vi "导出参数设置3.0.vi"(10 "输入":T1, 11 "路径":path) -> ()   [LabVIEW 2016]
uses:
  <vilib>/Utility/config.llb/Write Key (String).vi
  <vilib>/Utility/config.llb/Write Key (Double).vi
  <vilib>/Utility/config.llb/NI_LVConfig.lvlib
panel:
  in  "ESC":bool
  in  "OK":bool
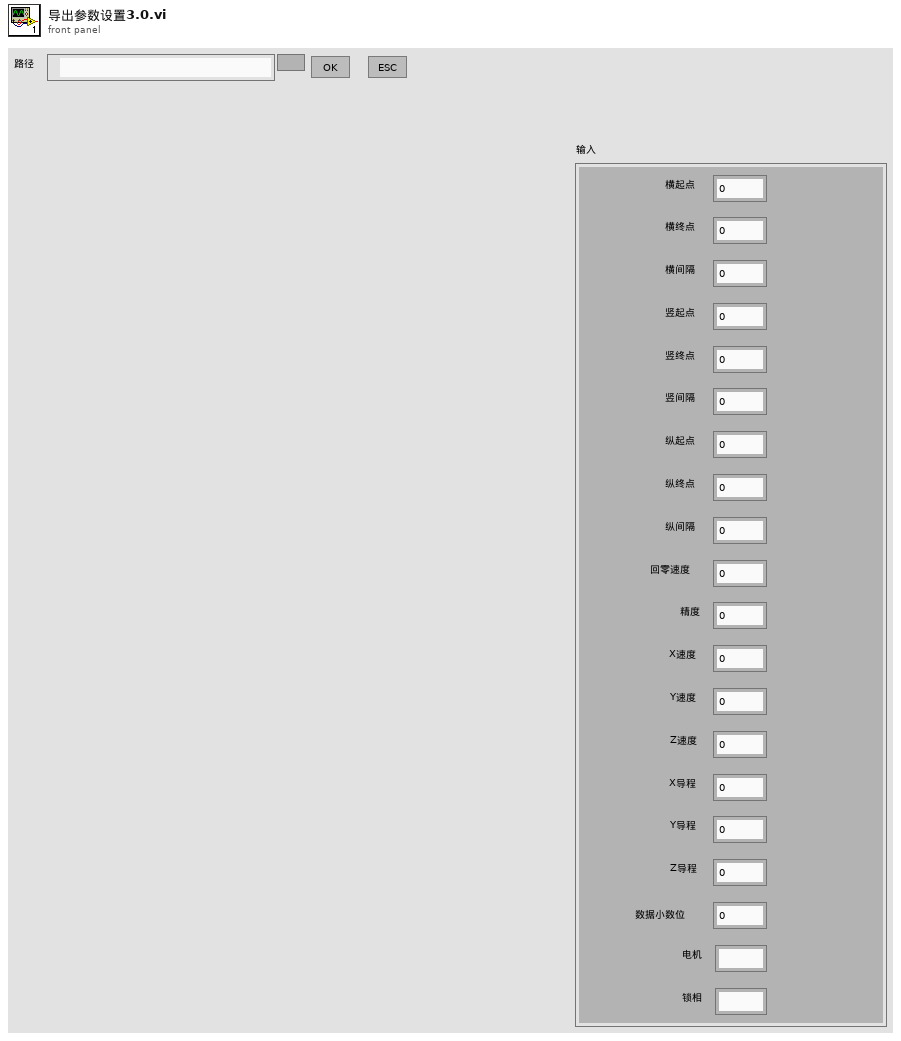
[diagram p1: front panel]
types:
  T1 = cluster{"横起点":dbl, "横终点":dbl, "横间隔":dbl, "竖起点":dbl, "竖终点":dbl, "竖间隔":dbl, "纵起点":dbl, "纵终点":dbl, "纵间隔":dbl, "回零速度":dbl, "精度":dbl, "X速度":dbl, "Y速度":dbl, "Z速度":dbl, "X导程":dbl, "Y导程":dbl, "Z导程":dbl, "数据小数位":dbl, "电机":string, "锁相":string}
  T2 = typedef "NI_LVConfig.lvlib/Config Data RefNum.ctl" = refnum<k1>
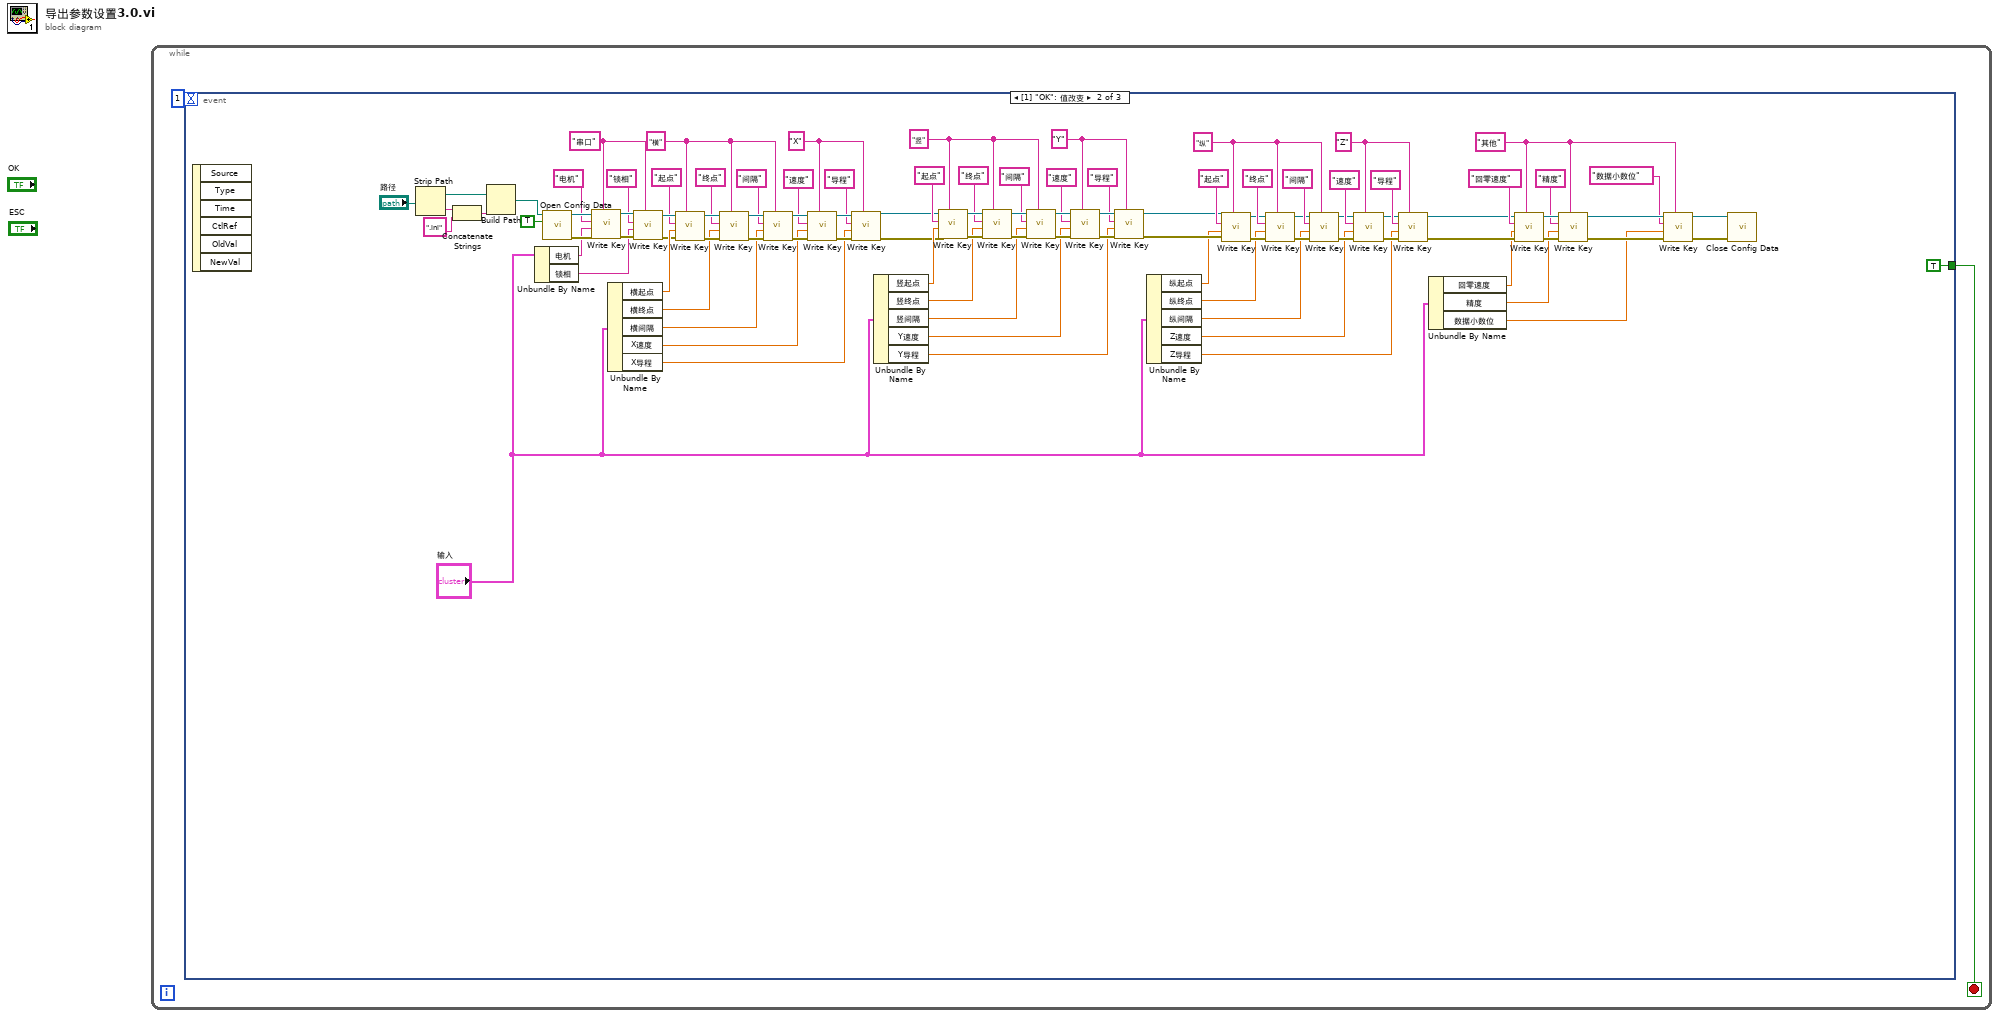
[diagram p0: block diagram]
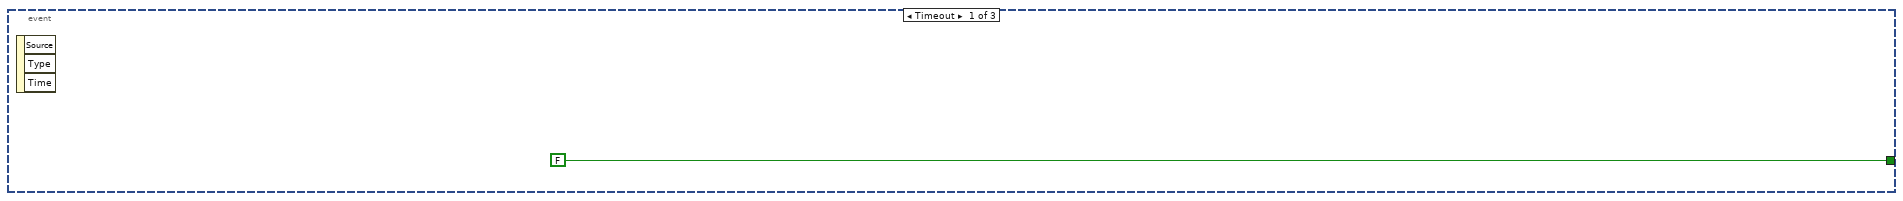
[diagram p2: hidden frame]
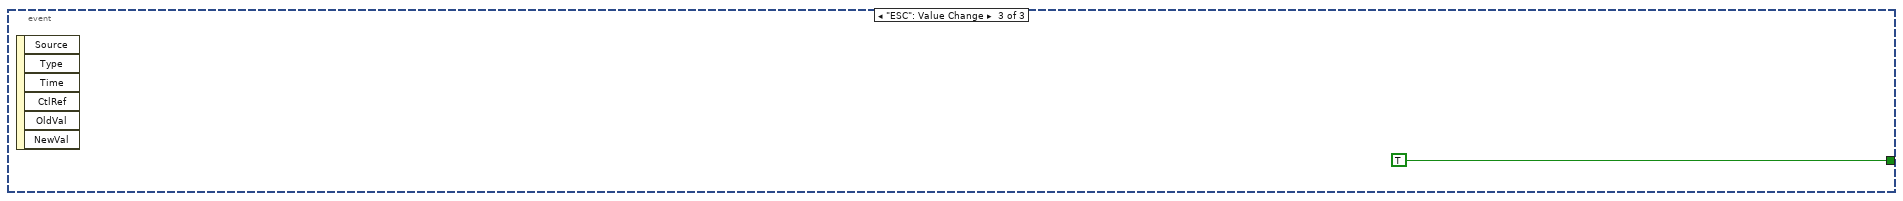
[diagram p3: hidden frame]
diagram:
  n1 = while {
    stop <- w1 stop-if-true
    n2 = event shown="[1] \"OK\": 值改变" {
      selector: _ -> [_ _ _]
      dyn-events: _ -> [_ _ _]
      timeout: 1 -> [_ _ _]
      tunnel: [FALSE TRUE TRUE] -> w1
      event Timeout {
        n3 = event-data() -> ()  [unwired: 1 in, 3 out]
      }
      event "OK": Value Change {
        w21 = "其他" ("section")
        w45 = "Y" ("section")
        w46 = "竖" ("section")
        w64 = "Z" ("section")
        w63 = "纵" ("section")
        w81 = "X" ("section")
        w87 = "横" ("section")
        w98 = "串口" ("section")
        n4 = event-data() -> ()  [unwired: 1 in, 6 out]
        n5 = Strip Path(path="路径") -> (stripped path=w8:path, name=w7:string)
        n6 = Concatenate Strings(w7, ".ini" ("字符串")) -> (w5:string)
        n7 = Build Path(base path=w8, name or relative path=w5) -> (appended path=w4:path)
        n8 = Unbundle By Name("输入") -> ("电机"=w85:string, "锁相"=w86:string)
        n9 = call <vilib>:"Open Config Data.vi"("create file if necessary (T)"=TRUE, "configuration file path"=w4) -> ("error out"=w93:errorcluster, "refnum"=w100:T2)  [unwired: 7 in, 1 out]
        n10 = call-poly <vilib>:"Write Key.vi"("section"=w98, "error in (no error)"=w93, "value"=w85, "key"="电机", "refnum"=w100) -> ("error out"=w92:errorcluster, "refnum out"=w99:T2)  [unwired: 4 in, 1 out]
        n11 = Unbundle By Name("输入") -> ("横起点"=w75:dbl, "横终点"=w73:dbl, "横间隔"=w72:dbl, "X速度"=w71:dbl, "X导程"=w70:dbl)
        n12 = call-poly <vilib>:"Write Key.vi"("section"=w98, "error in (no error)"=w92, "value"=w86, "key"="锁相", "refnum"=w99) -> ("error out"=w74:errorcluster, "refnum out"=w82:T2)  [unwired: 4 in, 1 out]
        n13 = call-poly <vilib>:"Write Key.vi"("section"=w87, "error in (no error)"=w74, "value"=w75, "key"="起点", "refnum"=w82) -> ("error out"=w97:errorcluster, "refnum out"=w96:T2)  [unwired: 4 in, 1 out]
        n14 = call-poly <vilib>:"Write Key.vi"("section"=w87, "error in (no error)"=w97, "value"=w73, "key"="终点", "refnum"=w96) -> ("error out"=w95:errorcluster, "refnum out"=w94:T2)  [unwired: 4 in, 1 out]
        n15 = call-poly <vilib>:"Write Key.vi"("section"=w87, "error in (no error)"=w95, "value"=w72, "key"="间隔", "refnum"=w94) -> ("error out"=w89:errorcluster, "refnum out"=w91:T2)  [unwired: 4 in, 1 out]
        n16 = call-poly <vilib>:"Write Key.vi"("section"=w81, "error in (no error)"=w89, "value"=w71, "key"="速度", "refnum"=w91) -> ("error out"=w88:errorcluster, "refnum out"=w90:T2)  [unwired: 4 in, 1 out]
        n17 = call-poly <vilib>:"Write Key.vi"("section"=w81, "error in (no error)"=w88, "value"=w70, "key"="导程", "refnum"=w90) -> ("error out"=w38:errorcluster, "refnum out"=w37:T2)  [unwired: 4 in, 1 out]
        n18 = Unbundle By Name("输入") -> ("竖起点"=w39:dbl, "竖终点"=w36:dbl, "竖间隔"=w35:dbl, "Y速度"=w34:dbl, "Y导程"=w33:dbl)
        n19 = call-poly <vilib>:"Write Key.vi"("section"=w46, "error in (no error)"=w38, "value"=w39, "key"="起点", "refnum"=w37) -> ("error out"=w54:errorcluster, "refnum out"=w53:T2)  [unwired: 4 in, 1 out]
        n20 = call-poly <vilib>:"Write Key.vi"("section"=w46, "error in (no error)"=w54, "value"=w36, "key"="终点", "refnum"=w53) -> ("error out"=w52:errorcluster, "refnum out"=w51:T2)  [unwired: 4 in, 1 out]
        n21 = call-poly <vilib>:"Write Key.vi"("section"=w46, "error in (no error)"=w52, "value"=w35, "key"="间隔", "refnum"=w51) -> ("error out"=w48:errorcluster, "refnum out"=w50:T2)  [unwired: 4 in, 1 out]
        n22 = call-poly <vilib>:"Write Key.vi"("section"=w45, "error in (no error)"=w48, "value"=w34, "key"="速度", "refnum"=w50) -> ("error out"=w47:errorcluster, "refnum out"=w49:T2)  [unwired: 4 in, 1 out]
        n23 = call-poly <vilib>:"Write Key.vi"("section"=w45, "error in (no error)"=w47, "value"=w33, "key"="导程", "refnum"=w49) -> ("error out"=w31:errorcluster, "refnum out"=w32:T2)  [unwired: 4 in, 1 out]
        n24 = Unbundle By Name("输入") -> ("纵起点"=w30:dbl, "纵终点"=w29:dbl, "纵间隔"=w28:dbl, "Z速度"=w27:dbl, "Z导程"=w26:dbl)
        n25 = call-poly <vilib>:"Write Key.vi"("section"=w63, "error in (no error)"=w31, "value"=w30, "key"="起点", "refnum"=w32) -> ("error out"=w55:errorcluster, "refnum out"=w56:T2)  [unwired: 4 in, 1 out]
        n26 = call-poly <vilib>:"Write Key.vi"("section"=w63, "error in (no error)"=w55, "value"=w29, "key"="终点", "refnum"=w56) -> ("error out"=w57:errorcluster, "refnum out"=w58:T2)  [unwired: 4 in, 1 out]
        n27 = call-poly <vilib>:"Write Key.vi"("section"=w63, "error in (no error)"=w57, "value"=w28, "key"="间隔", "refnum"=w58) -> ("error out"=w61:errorcluster, "refnum out"=w59:T2)  [unwired: 4 in, 1 out]
        n28 = call-poly <vilib>:"Write Key.vi"("section"=w64, "error in (no error)"=w61, "value"=w27, "key"="速度", "refnum"=w59) -> ("error out"=w62:errorcluster, "refnum out"=w60:T2)  [unwired: 4 in, 1 out]
        n29 = call-poly <vilib>:"Write Key.vi"("section"=w64, "error in (no error)"=w62, "value"=w26, "key"="导程", "refnum"=w60) -> ("error out"=w16:errorcluster, "refnum out"=w17:T2)  [unwired: 4 in, 1 out]
        n30 = Unbundle By Name("输入") -> ("回零速度"=w15:dbl, "精度"=w14:dbl, "数据小数位"=w13:dbl)
        n31 = call-poly <vilib>:"Write Key.vi"("section"=w21, "error in (no error)"=w16, "value"=w15, "key"="回零速度", "refnum"=w17) -> ("error out"=w25:errorcluster, "refnum out"=w24:T2)  [unwired: 4 in, 1 out]
        n32 = call-poly <vilib>:"Write Key.vi"("section"=w21, "error in (no error)"=w25, "value"=w14, "key"="精度", "refnum"=w24) -> ("error out"=w23:errorcluster, "refnum out"=w22:T2)  [unwired: 4 in, 1 out]
        n33 = call-poly <vilib>:"Write Key.vi"("section"=w21, "error in (no error)"=w23, "value"=w13, "key"="数据小数位", "refnum"=w22) -> ("error out"=w12:errorcluster, "refnum out"=w11:T2)  [unwired: 4 in, 1 out]
        n34 = call <vilib>:"Close Config Data.vi"("error in (no error)"=w12, "refnum"=w11) -> ()  [unwired: 8 in, 2 out]
      }
      event "ESC": Value Change {
        n35 = event-data() -> ()  [unwired: 1 in, 6 out]
      }
    }
  }
